vi "Subvi pixelclock.vi"(9 "Lineclock":bool) -> (2 "PixelclockChange":bool, 6 "PixelclockMon":bool)   [LabVIEW 2017]
uses:
  <vilib>/rvi/Emulation/niFpgaSctlEmulationGetInTimedLoop.vi
  GV N pixelclock per line.vi
  <vilib>/rvi/Memory/Memory_Emulation/nirvimemoryFastEmulation.vi
  <vilib>/rvi/Memory/Memory_Emulation/nirvimemoryEmulation.vi
  <vilib>/rvi/Emulation/niFpgaEmulationIsFPGAContextNoSignature.vi
  <vilib>/rvi/DataTransferAndStorage/Container/Common/niFpgaContainerGetUniqueNameForEmu.vi
  <vilib>/rvi/Emulation/niFpgaProcessEmulError.vi
  <vilib>/rvi/errors/nirviReportUnexpectedCaseInternalError (U32).vi
  GV FIFOOUT gate.vi
  <vilib>/rvi/DataTransferAndStorage/Container/XNode/niFpgaContainer.xnode
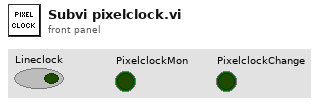
[diagram p1: front panel]
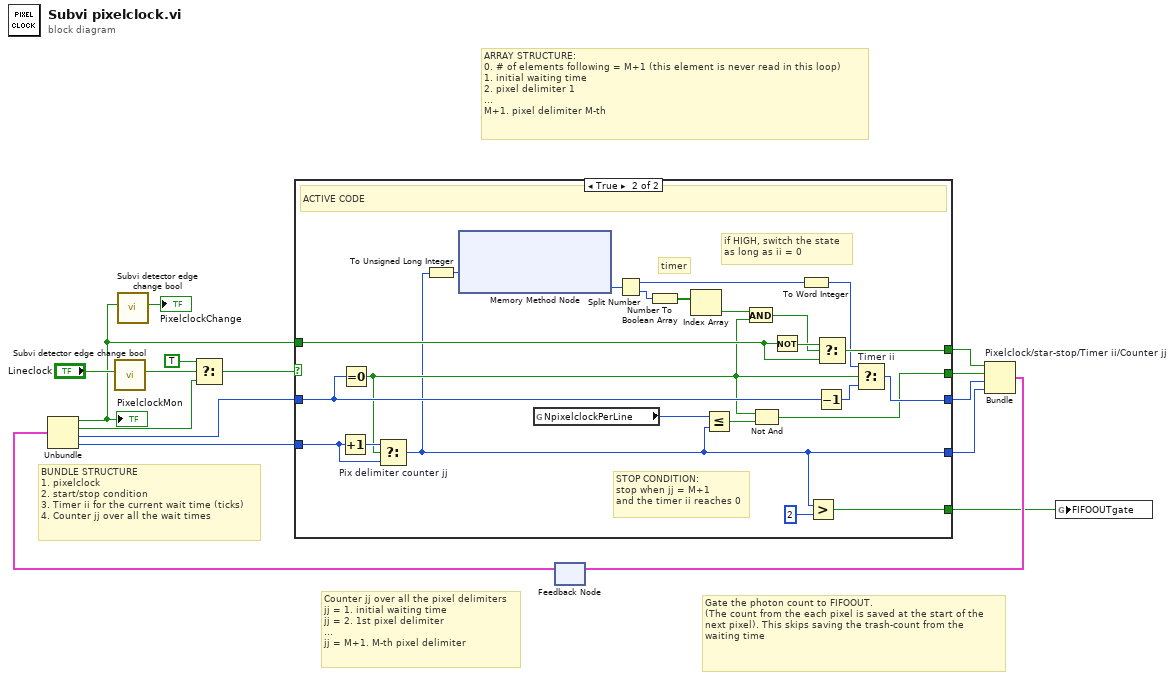
[diagram p0: block diagram]
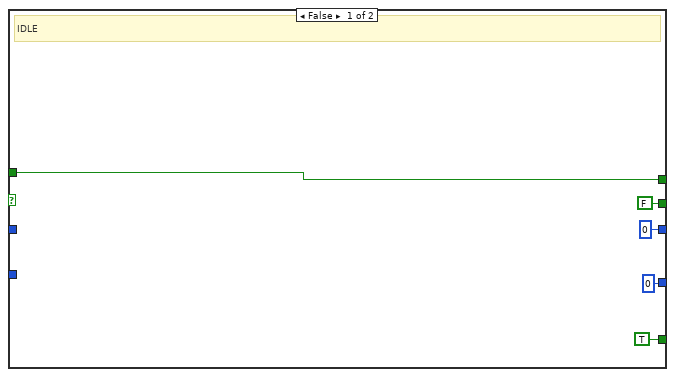
[diagram p2: hidden frame]
diagram:
  # "Counter jj over all the pixel delimiters\njj = 1. initial waiting time\njj = 2. 1st pixel delimiter\n...\njj = M+1. M-th pixel delimiter"
  # "Gate the photon count to FIFOOUT.\n(The count from the each pixel is saved at the start of the\nnext pixel). This skips saving the trash-count from the\nwaiting time"
  # "BUNDLE STRUCTURE\n1. pixelclock\n2. start/stop condition\n3. Timer ii for the current wait time (ticks)\n4. Counter jj over all the wait times"
  # "ARRAY STRUCTURE:\n0. # of elements following = M+1 (this element is never read in this loop)\n1. initial waiting time \n2. pixel delimiter 1\n...\nM+1. pixel delimiter M-th"
  n1 = call "Subvi detector edge change bool.vi"("Input"="Lineclock") -> ("Output"=w4:bool)  [unwired: 8 in]
  n2 = feedback #1() -> (w10:cluster{bool, bool, i16, i16})  [unwired: 1 in]
  n3 = Unbundle(w10) -> (w2:bool, w8:bool, w7:i16, w6:i16)
  "PixelclockMon" <- w2
  n4 = call "Subvi detector edge change bool.vi"("Input"=w2) -> ("Output"=→"PixelclockChange":bool)  [unwired: 8 in]
  n5 = Select(t=TRUE, s=w4, f=w8) -> (s? t:f=w16:bool)
  n6 = case shown="True" w16 {
    tunnel: [FALSE w27] -> w14
    tunnel: w7 -> [_ w36]
    tunnel: [i16 0 w39] -> w13
    tunnel: [w19 w40] -> w9
    tunnel: w2 -> [w19 w37]
    tunnel: w6 -> [_ w35]
    tunnel: [i16 0 w26] -> w12
    tunnel: [TRUE w24] -> w5
    frame False {
      # "IDLE"
    }
    frame True {
      # "STOP CONDITION:\nstop when jj = M+1\nand the timer ii reaches 0"
      # "timer"
      # "if HIGH, switch the state\nas long as ii = 0"
      # "ACTIVE CODE"
      n7 = Increment(x=w35) -> (x+1=w44:i16)
      n8 = Equal To 0?(x=w36) -> (x = 0?=w30:bool)
      n9 = Select "Pix delimiter counter jj"(t=w44, s=w30, f=w35) -> (s? t:f=w26:i16)
      n10 = To Unsigned Long Integer(number=w26) -> (unsigned 32bit integer=w28:u32)
      n11 = xnode ("Memory Method Node")("Address"=w28) -> ("Data"=w29:u32)  [unwired: 1 in, 1 out]
      n12 = global read "GV N pixelclock per line.vi" "NpixelclockPerLine"() -> (w23:i16)
      n13 = Split Number(x=w29) -> (hi(x)=w38:u16, lo(x)=w42:u16)
      n14 = Number To Boolean Array(number=w42) -> (Boolean array=w43:bool[])
      n15 = Index Array(array=w43) -> (element=w31:bool)  [unwired: 1 in]
      n16 = Less Or Equal?(x=w23, y=w26) -> (x <= y?=w33:bool)
      n17 = And(x=w31, y=w30) -> (x .and. y?=w32:bool)
      n18 = Not And(1:w33, 2:w30) -> (0:w27:bool)
      n19 = Not(x=w37) -> (.not. x?=w41:bool)
      n20 = To Word Integer(number=w38) -> (16bit integer=w22:i16)
      n21 = Greater?(x=w26, y=i16 2) -> (0:w24:bool)
      n22 = Decrement(x=w36) -> (x-1=w34:i16)
      n23 = Select(t=w41, s=w32, f=w37) -> (s? t:f=w40:bool)
      n24 = Select "Timer ii"(t=w22, s=w30, f=w34) -> (s? t:f=w39:i16)
    }
  }
  n25 = Bundle "Pixelclock/star-stop/Timer ii/Counter jj"(w9, w14, w13, w12) -> (w11:cluster{bool, bool, i16, i16})  [unwired: 1 in]
  n26 = feedback-in #1(w11) -> ()
  n27 = global write "GV FIFOOUT gate.vi" "FIFOOUTgate"(w5) -> ()
